vi "marshalling.vi"(8 "error in (no error)":errorcluster, 10 "Variant":variant, 11 "Serializer":refnum<class "Serializer.JDP-JSON.lvclass">) -> (0 "error out":errorcluster, 2 "JSON String":string, 3 "Serializer out":refnum<class "Serializer.JDP-JSON.lvclass">)   [LabVIEW 2019, in "OpenSerializer.JDP-JSON.lvlib" / "Serializer.JDP-JSON.lvclass"]
uses:
  Serializer.JDP-JSON.lvclass
  Serializer.JDP-JSON.lvclass/Serializer.JDP-JSON.ctl
  <vilib>/JDP Science/JSONtext/JSONtext.lvlib
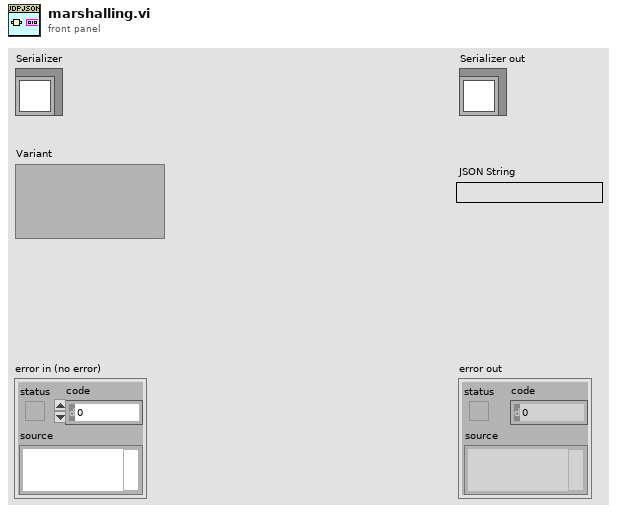
[diagram p1: front panel]
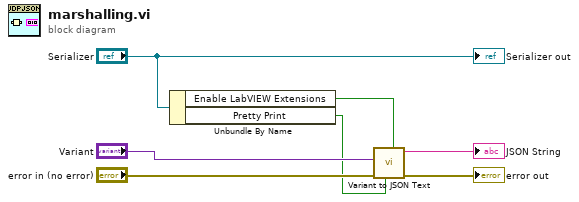
[diagram p0: block diagram]
diagram:
  n1 = Unbundle By Name("Serializer") -> ("Enable LabVIEW Extensions"=w2:bool, "Pretty Print"=w1:bool)
  n2 = call <vilib>:"Variant to JSON Text.vi"("enable LabVIEW extensions? (T)"=w2, "Pretty Print?"=w1, "error in (no error)"="error in (no error)", "Variant"="Variant") -> ("error out"=→"error out":errorcluster, "<JSON>"=→"JSON String":string)  [unwired: 5 in, 1 out]
  "Serializer out" <- "Serializer"
